vi "Enable Display.vi"(8 "error in (no error)":errorcluster, 9 "String to Show (\"\")":string, 10 "Enable Display (T: Enable)":bool=TRUE, 11 "VISA resource name":refnum<visa-resource-name>) -> (0 "error out":errorcluster, 3 "VISA resource name out":refnum<visa-resource-name>)   [LabVIEW 2019, in "Agilent 3352X Series.lvlib"]
doc: "Disables or enables the waveform generator front-panel display. When it is disabled, the front-panel display is blacked and a specified string is shown in the center of the screen.\n\n<b>Note</b>:\n(1) This VI does not check the instrument status."
uses:
  Agilent 3352X Series.lvlib
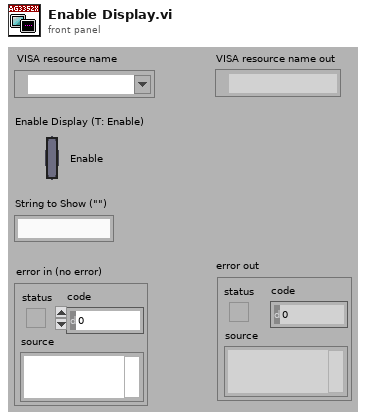
[diagram p1: front panel]
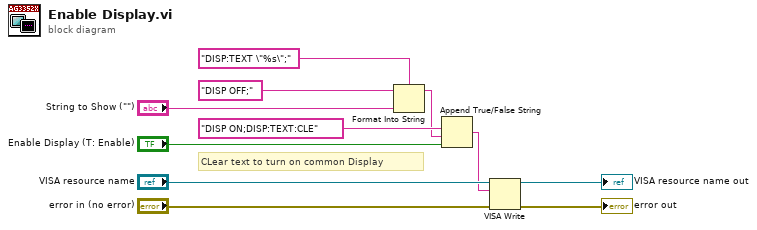
[diagram p0: block diagram]
diagram:
  # "CLear text to turn on common Display"
  n1 = Format Into String(format string="DISP:TEXT \"%s\";", initial string="DISP OFF;", "String to Show (\"\")") -> (resulting string=w3:string)  [unwired: 1 in, 1 out]
  n2 = Append True/False String(1:"Enable Display (T: Enable)", 2:w3, 3:"DISP ON;DISP:TEXT:CLE") -> (0:w5:string)  [unwired: 1 out]
  n3 = VISA Write(VISA resource name="VISA resource name", write buffer=w5, error in (no error)="error in (no error)") -> (VISA resource name out=→"VISA resource name out":refnum<visa-resource-name>, error out=→"error out":errorcluster)  [unwired: 1 out]
